vi "vlcd.vi"() -> ()   [LabVIEW 2017]
panel:
  in  "stop":bool
  in  "buffer":u8[](array[numeric])
  in  "LCD EMULATOR(":bool[][](array[boolean])
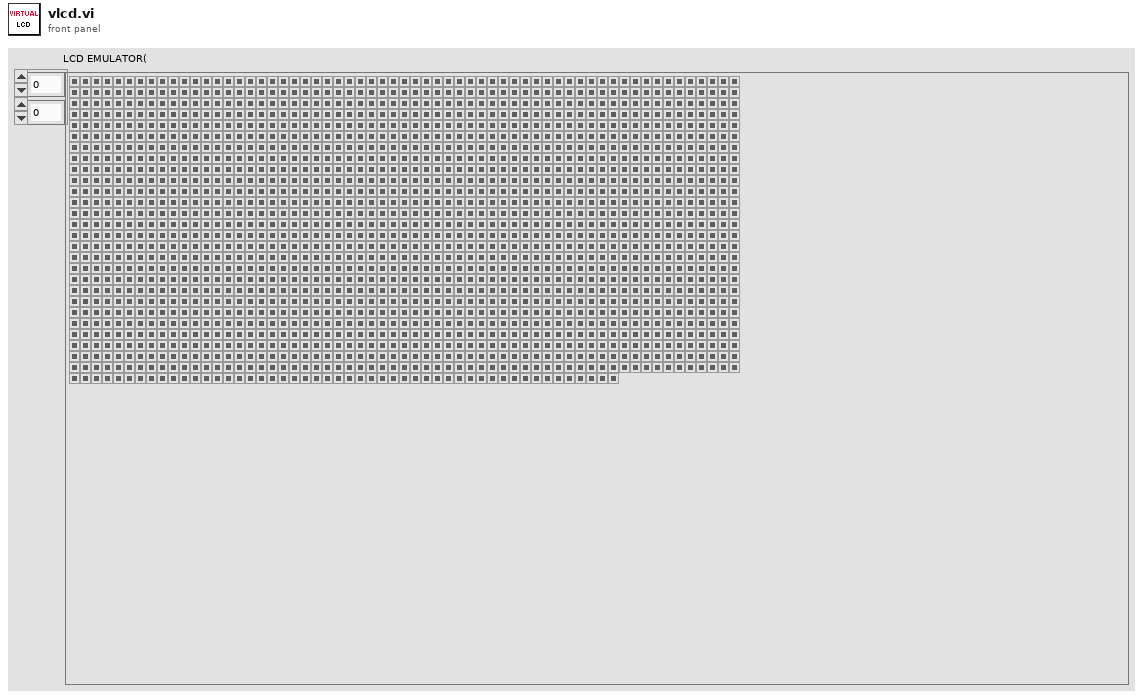
[diagram p1: front panel]
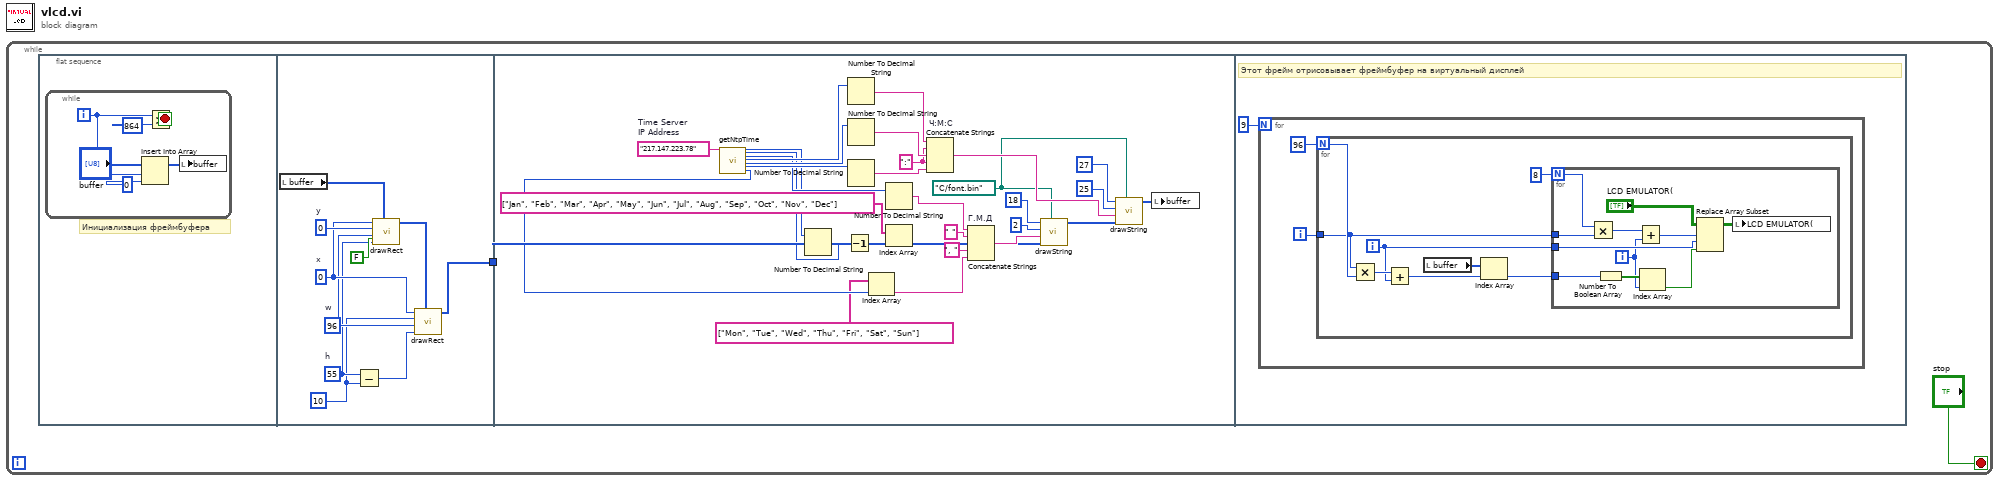
[diagram p0: block diagram]
diagram:
  n1 = while {
    stop <- "stop" stop-if-true
    n2 = flat-sequence {
      tunnel: [w9] -> w1
      tunnel: w1 -> [w31]
      frame #0 {
        # "Инициализация фреймбуфера"
        n3 = while {
          i -> [w3]
          stop <- w5 stop-if-true
          n4 = Insert Into Array(array="buffer", index=w3, new element=u8 0 ("new element/subarray")) -> (w8:u8[])
          n5 = Greater?(x=w3, y=864 ("x")) -> (0:w5:bool)
          n6 = local write "buffer"(w8) -> ()
        }
      }
      frame #1 {
        w12 = u8 10 ("y")
        w13 = u8 55  # h
        w14 = u8 96  # w
        w17 = u8 0  # y
        w15 = u8 0  # x
        n7 = local read "buffer"() -> (w18:u8[])
        n8 = Subtract(x=w13, y=w12) -> (x-y=w11:u8)
        n9 = call "drawRect.vi"("fill"=FALSE ("filled or not"), "input_buffer"=w18, "h"=w13, "w"=w14, "y"=w17, "x"=w15) -> ("output_buffer"=w10:u8[])  [unwired: 5 in]
        n10 = call "drawRect.vi"("input_buffer"=w10, "h"=w11, "w"=w14, "y"=w12, "x"=w15) -> ("output_buffer"=w9:u8[])  [unwired: 6 in]
      }
      frame #2 {
        w33 = path "C:/font.bin" ("file")
        w43 = ":" ("string")
        w48 = "217.147.223.78"  # Time Server IP Address
        n11 = call "getNtpTime.vi"("Time Server\nIP Address"=w48) -> ("year"=w28:i32, "month"=w26:i32, "day of month"=w30:i32, "hour"=w42:i32, "minute"=w41:i32, "second"=w40:i32, "day of week"=w23:i32)  [unwired: 19 in, 1 out]
        n12 = Number To Decimal String(number=w28) -> ()  [unwired: 1 in, 1 out]
        n13 = Decrement(x=w26) -> (x-1=w27:i32)
        n14 = Number To Decimal String(number=w42) -> (decimal integer string=w46:string)  [unwired: 1 in]
        n15 = Number To Decimal String(number=w41) -> (decimal integer string=w45:string)  [unwired: 1 in]
        n16 = Number To Decimal String(number=w40) -> (decimal integer string=w44:string)  [unwired: 1 in]
        n17 = Index Array(array=string[] ["Mon", "Tue", "Wed", "Thu", "Fri", "Sat", "Sun"], index=w23) -> (element=w20:string)
        n18 = Number To Decimal String(number=w30) -> (decimal integer string=w29:string)  [unwired: 1 in]
        n19 = Index Array(array=string[] ["Jan", "Feb", "Mar", "Apr", "May", "Jun", "Jul", "Aug", "Sep", "Oct", "Nov", "Dec"], index=w27) -> (element=w25:string)
        n20 = Concatenate Strings "Ч:М:С"(w46, w43, w45, w43, w44) -> (w39:string)
        n21 = Concatenate Strings "Г.М.Д"(w29, " " ("string"), w25, ", " ("string"), w20) -> (w47:string)
        n22 = call "drawString.vi"("font file"=w33, "input buffer"=w31, "input string"=w47, "y"=u8 2, "x"=u8 18) -> ("output buffer"=w38:u8[])  [unwired: 5 in, 1 out]
        n23 = call "drawString.vi"("font file"=w33, "input buffer"=w38, "input string"=w39, "y"=u8 25, "x"=u8 27) -> ("output buffer"=w32:u8[])  [unwired: 5 in, 1 out]
        n24 = local write "buffer"(w32) -> ()
      }
      frame #3 {
        # "Этот фрейм отрисовывает фреймбуфер на виртуальный дисплей"
        n25 = for {
          N: 9 -> [_]
          i -> [w50]
          n26 = for {
            N: 96 -> [w59]
            tunnel: w50 -> [w52]
            i -> [w53]
            n27 = Multiply(x=w52, y=w59) -> (x*y=w58:i32)
            n28 = Add(x=w58, y=w53) -> (x+y=w54:i32)
            n29 = local read "buffer"() -> (w56:u8[])
            n30 = Index Array(array=w56, index=w54) -> (element=w55:u8)
            n31 = for {
              N: 8 -> [w63]
              tunnel: w55 -> [w67]
              tunnel: w53 -> [w66]
              tunnel: w52 -> [w62]
              i -> [w65]
              n32 = Multiply(x=w63, y=w62) -> (x*y=w61:i32)
              n33 = Number To Boolean Array(number=w67) -> (Boolean array=w68:bool[])
              n34 = Add(x=w61, y=w65) -> (x+y=w64:i32)
              n35 = Index Array(array=w68, index=w65) -> (element=w70:bool)
              n36 = Replace Array Subset(array="LCD EMULATOR(", new element=w70, index (row)=w64, index (col)=w66) -> (w69:bool[][])
              n37 = local write "LCD EMULATOR("(w69) -> ()
            }
          }
        }
      }
    }
  }
